vi "ElevatorSpecificHeightSendCmd.vi"(0 "SpecHeightStage3":dbl, 1 "SpecHeightOuter":dbl, 3 "error in (no error)":errorcluster) -> (10 "error out":errorcluster)   [LabVIEW 2023]
doc: "Sets the height demand by writing the input to the ElevatorCmdSpecificHeight Global and then sending a boolean command to the boolean receive called \"ElevSpecHeight\" (in ElevatorExecuteLogic.vi)\n\nInputs:\n--SpecHeight--numeric--inches\n--error in\nOuputs:\n--error out"
uses:
  <vilib>/Rock Robotics/WPI/ThirdParty/JAS_Junk/TrajLib/VI/BoolCmd_Send_Internal.vi
  <vilib>/Rock Robotics/WPI/ThirdParty/JAS_Junk/TrajLib/VI/BoolCmd_ObtainQueue.vi
  ElevatorGlobal.vi
  <vilib>/Rock Robotics/WPI/ThirdParty/JAS_Junk/TrajLib/Trajectory_Library.lvlib
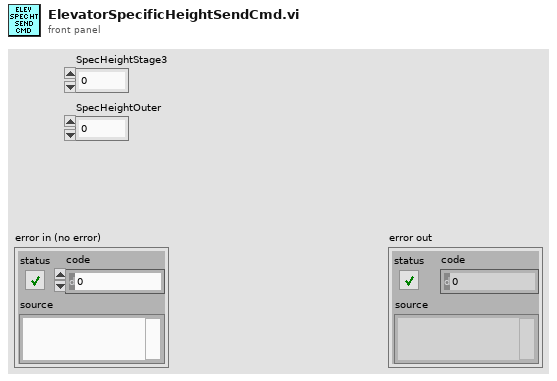
[diagram p1: front panel]
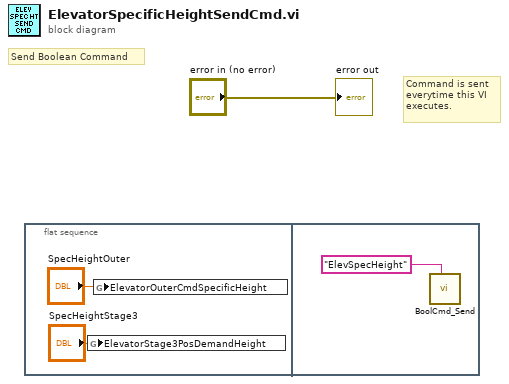
[diagram p0: block diagram]
diagram:
  # "Command is sent\neverytime this VI\nexecutes."
  # "Send Boolean Command"
  n1 = flat-sequence {
    frame #0 {
      n2 = global write "ElevatorGlobal.vi" "ElevatorStage3PosDemandHeight"("SpecHeightStage3") -> ()
      n3 = global write "ElevatorGlobal.vi" "ElevatorOuterCmdSpecificHeight"("SpecHeightOuter") -> ()
    }
    frame #1 {
      n4 = call <vilib>:"BoolCmd_Send.vi"("Command Name"="ElevSpecHeight") -> ()  [unwired: 10 in, 1 out]
    }
  }
  "error out" <- "error in (no error)"
